vi "Abort Client Loop.vi"(8 "error in (no error)":errorcluster, 11 "VISA Client in":refnum<class "Serial Client.lvclass">) -> (0 "error out":errorcluster, 3 "VISA Client out":refnum<class "Serial Client.lvclass">)   [LabVIEW 2020, in "Stream-Serial.lvlib" / "Serial Client.lvclass"]
uses:
  Serial Client.lvclass
  C:/Program Files (x86)/National Instruments/LabVIEW 2020/vi.lib/IlluminatedG/lv-stream/Connection/Connection.lvclass
  <vilib>/IlluminatedG/lv-stream/Connection/State.ctl
  Serial Client.lvclass/Serial Client.ctl
  <vilib>/IlluminatedG/lv-stream/Connection/Connection.lvclass
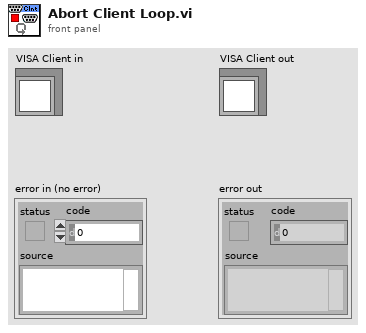
[diagram p1: front panel]
types:
  T1 = typedef "Stream.lvlib/Connection.lvclass/State.ctl" = enum16{"Closed", "Idle", "Connecting", "Connected", "Shutdown"}
  T2 = typedef "Stream-Serial.lvlib/Serial Client.lvclass/Ref Data.ctl" = cluster{"Stream":refnum<class "Serial Stream.lvclass">, "Client Loop":refnum<vi>, "Port Config":T3, "VISA Resource":refnum<visa-resource-name>}
  T3 = typedef "Stream-Serial.lvlib/Serial Client.lvclass/Port Config.ctl" = cluster{"Baud (115200)":u32, "Data Bits (8)":u8, "Stop Bits (1)":T4, "Flow Control":T5, "Use LineTerm?":bool, "LineTerm (\\n)":string, "Timeout ms (10000)":i32, "Parity (None)":T6}
  T4 = typedef "Stream-Serial.lvlib/Serial Client.lvclass/Stop Bits.ctl" = u16
  T5 = typedef "Stream-Serial.lvlib/Serial Client.lvclass/Flow Control.ctl" = u16
  T6 = typedef "Stream-Serial.lvlib/Serial Client.lvclass/Parity.ctl" = enum16{"None", "Odd", "Even", "Mark", "Space"}
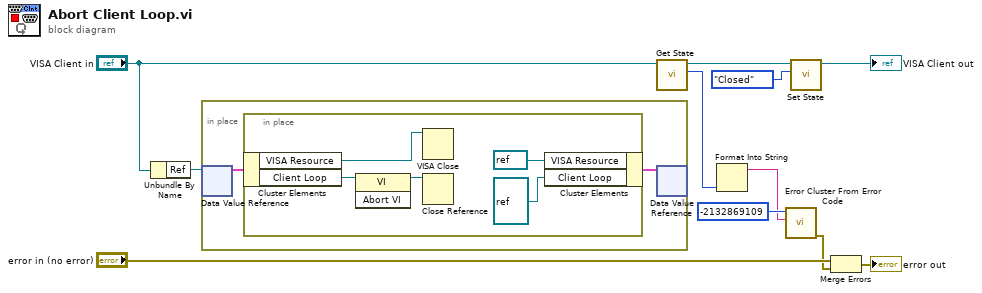
[diagram p0: block diagram]
diagram:
  n1 = Unbundle By Name("VISA Client in") -> ("Ref"=w10:refnum<data-value>)
  n2 = in-place {
    n3 = in-place-dvr #1(w10) -> (w13:T2)  [unwired: 1 out]
    n4 = in-place {
      n5 = in-place-cluster #2(w13) -> ("VISA Resource"=w16:refnum<visa-resource-name>, "Client Loop"=w18:refnum<vi>)
      n6 = invoke class="VI" method="Abort VI"(reference=w18) -> (reference out=w17:refnum<vi>)  [unwired: 2 in, 2 out]
      n7 = VISA Close(VISA resource name=w16) -> ()  [unwired: 1 in, 1 out]
      n8 = Close Reference(reference=w17) -> ()  [unwired: 1 in, 1 out]
      n9 = in-place-cluster #2("VISA Resource"=refnum<visa-resource-name> refnum, "Client Loop"=refnum<vi> refnum) -> (w12:T2)
    }
    n10 = in-place-dvr #1(w12) -> ()  [unwired: 2 out]
  }
  n11 = call <vilib>:"Get State.vi"("Connection in"="VISA Client in") -> ("State"=w4:T1, "Connection out"=w3:refnum<class "Serial Client.lvclass">)  [unwired: 8 in, 1 out]
  n12 = Format Into String(w4) -> (resulting string=w8:string)  [unwired: 3 in, 1 out]
  n13 = call <vilib>:"Error Cluster From Error Code.vi"("error message (\"\")"=w8, "error code (0)"=-2132869109) -> ("error out"=w6:errorcluster)  [unwired: 7 in]
  n14 = call <vilib>:"Set State.vi"("State"=State."Closed", "Connection in"=w3) -> ("Connection out"=→"VISA Client out":refnum<class "Serial Client.lvclass">)  [unwired: 8 in, 1 out]
  n15 = Merge Errors("error in (no error)", w6) -> (→"error out":errorcluster)
